vi "Serial  send and receive.vi"(6 "Read Timeout Value":u32=500, 7 "读取字节总数":u32=1, 8 "error in (no error)":errorcluster caption="错误输入（无错误）", 9 "读取":bool, 10 "command":u8[](array[numeric]) format="%02x", 11 "VISA IN":refnum<visa-resource-name>="COM1" caption="serial number") -> (0 "error out":errorcluster caption="错误输出", 1 "Command":string, 2 "read buffer":string, 3 "VISA OUT":refnum<visa-resource-name>, 5 "Send/Read":string)   [LabVIEW 2013]
uses:
  <vilib>/Instr/_visa.llb/VISA Configure Serial Port (Instr).vi
panel:
  in  "baud rate":u32=115200
  out "Number of Bytes at Serial Port":u32
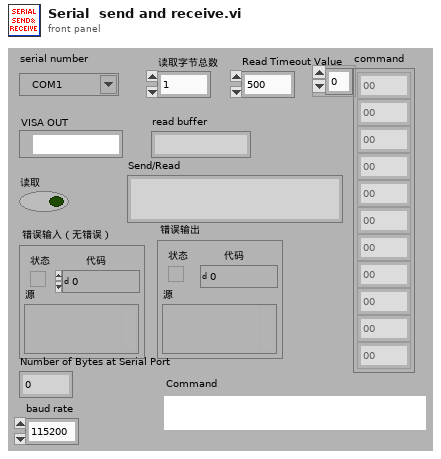
[diagram p1: front panel]
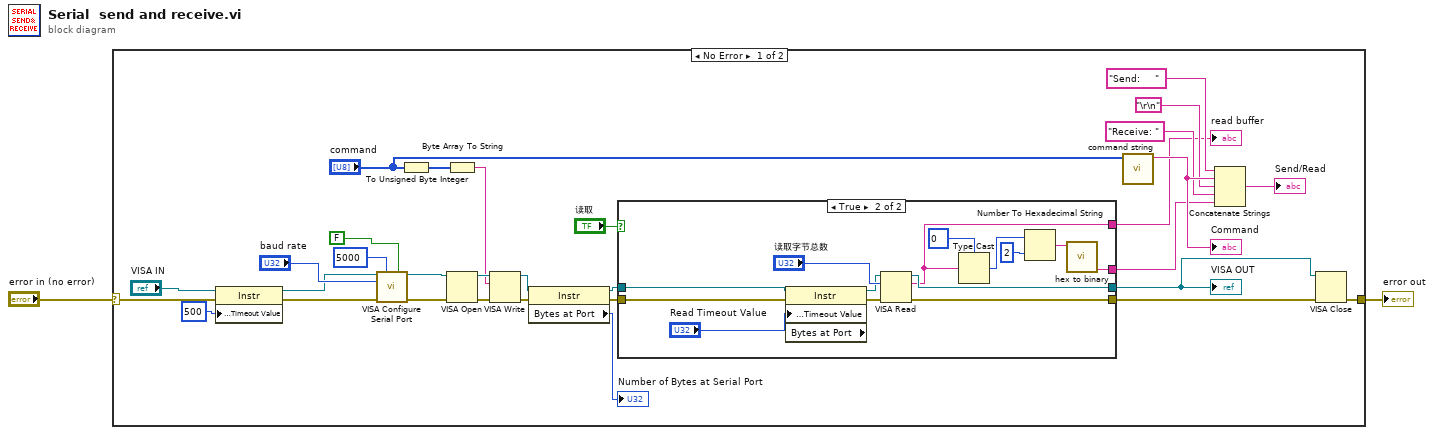
[diagram p0: block diagram]
diagram:
  n1 = case shown="No Error" "error in (no error)" {
    selector: "error in (no error)" -> [w21 w50]
    tunnel: [w19 w50] -> w1
    frame No Error {
      n2 = property class="Instr"(reference="VISA IN", error in=w21, "General Settings:Timeout Value"=u32 500) -> (reference out=w23:refnum<visa-resource-name>, error out=w22:errorcluster)
      n3 = call-poly "VISA Configure Serial Port"("VISA resource name"=w23, "timeout (10sec)"=u32 5000, "Enable Termination\nChar (T)"=FALSE ("Enable Termination\nChar (T)"), "baud rate (9600)"="baud rate", "error in (no error)"=w22) -> ("VISA resource name out"=w30:refnum<visa-resource-name>, "error out"=w31:errorcluster)  [unwired: 3 in, 6 out]
      n4 = To Unsigned Byte Integer(number="command") -> (unsigned 8bit integer=w27:u8[])
      n5 = Byte Array To String(unsigned byte array=w27) -> (string=w28:string)
      n6 = VISA Open(error in (no error)=w31, VISA resource name=w30) -> (VISA resource name=w32:refnum<visa-resource-name>, error out=w33:errorcluster)  [unwired: 3 out]
      n7 = VISA Write(VISA resource name=w32, write buffer=w28, error in (no error)=w33) -> (VISA resource name out=w15:refnum<visa-resource-name>, error out=w13:errorcluster)  [unwired: 1 out]
      n8 = property class="Instr"(reference=w15, error in=w13) -> (reference out=w14:refnum<visa-resource-name>, error out=w12:errorcluster, "Bytes at Port"=→"Number of Bytes at Serial Port":u32)
      n9 = case shown="True" "读取" {
        tunnel: w12 -> [w34 w48]
        tunnel: w14 -> [w35 w47]
        tunnel: [w35 w43] -> w18
        tunnel: [w34 w42] -> w17
        tunnel: [_ w39] -> w4
        tunnel: [_ w36] -> w3
        frame False {
        }
        frame True {
          n10 = property class="Instr" props=["General Settings:Timeout Value", "Bytes at Port"](reference=w47, error in=w48, "General Settings:Timeout Value"="Read Timeout Value") -> (reference out=w46:refnum<visa-resource-name>, error out=w45:errorcluster)  [unwired: 1 out]
          n11 = VISA Read(VISA resource name=w46, byte count="读取字节总数", error in (no error)=w45) -> (VISA resource name out=w43:refnum<visa-resource-name>, read buffer=w39:string, error out=w42:errorcluster)  [unwired: 1 out]
          n12 = Type Cast(type=u8 0 ("字节总数"), x=w39) -> (*(type *) &x=w41:u8)
          n13 = Number To Hexadecimal String(1:i16 2 ("宽度(-)"), 2:w41) -> (0:w37:string)
          n14 = call "hex to binary.vi"("字符串"=w37) -> ("Result"=w36:string)  [unwired: 9 in, 1 out]
        }
      }
      "VISA OUT" <- w18
      "read buffer" <- w4
      n15 = call "command string.vi"("DATA"="command") -> ("Command"=w8:string)  [unwired: 10 in]
      "Command" <- w8
      n16 = Concatenate Strings("Send:     " ("字符串"), w8, "\r\n", "Receive: " ("字符串"), w3) -> (→"Send/Read":string)
      n17 = VISA Close(VISA resource name=w18, error in (no error)=w17) -> (error out=w19:errorcluster)
    }
    frame Error {
    }
  }
  "error out" <- w1
